vi "Configure Channel Delay.vi"(0 "Digital Delay Generator in":refnum<class "Digital Delay Generator.lvclass">, 5 "Target Channel":T1, 7 "Reference Channel":T1, 9 "Delay (s)":dbl, 11 "error in (no error)":errorcluster) -> (4 "Digital Delay Generator out":refnum<class "Digital Delay Generator.lvclass">, 15 "error out":errorcluster)   [LabVIEW 2018, in "Digital Delay Generator.lvlib" / "Digital Delay Generator.lvclass"]
uses:
  Digital Delay Generator.lvclass
  Custom Controls/Channel.ctl
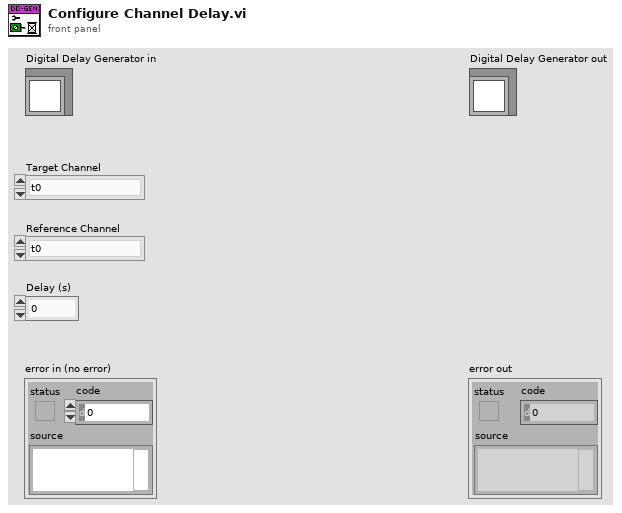
[diagram p1: front panel]
types:
  T1 = typedef "Digital Delay Generator.lvlib/Digital Delay Generator.lvclass/Channel.ctl" = enum16{"t0", "A", "B", "C", "D", "E", "F", "G", "H"}
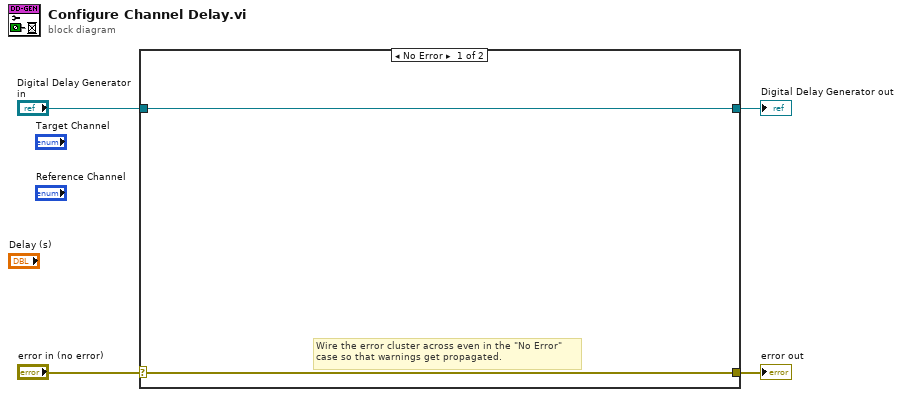
[diagram p0: block diagram]
diagram:
  n1 = case shown="No Error" "error in (no error)" {
    selector: "error in (no error)" -> [w5 w8]
    tunnel: [w5 w8] -> w3
    tunnel: [w6 w7] -> w1
    tunnel: "Digital Delay Generator in" -> [w6 w7]
    frame No Error {
      # "Wire the error cluster across even in the \"No Error\"\ncase so that warnings get propagated."
    }
    frame Error {
    }
  }
  "error out" <- w3
  "Digital Delay Generator out" <- w1
